vi "Retro.vi"(11 "Choose Directory":path) -> ()   [LabVIEW 2022 SP3]
uses:
  <vilib>/Analysis/NI_AALPro.lvlib
  <vilib>/Analysis/2dsp.llb/Complex FFT.vi
  <vilib>/Analysis/3filter.llb/Filter Passband Type.ctl
  <vilib>/Analysis/NI_AALBase.lvlib
  <vilib>/Analysis/3filter.llb/Butterworth Filter (DBL).vi
  <vilib>/Analysis/baseanly.llb/Quick Scale 1D.vi
  <vilib>/Analysis/baseanly.llb/Mean (DBL).vi
panel:
  in  "Save Directory":path
  out "Intensity Graph 3":sgl[][](graph)
  out "EKG 3":dbl[](graph)
  out "EKG 2":dbl[](graph)
  out "Intensity Graph 2":dbl[][](graph)
  in  "Use Selected Files":bool
  in  "Listbox":i32[](listbox)
  in  "file ext":string="000"
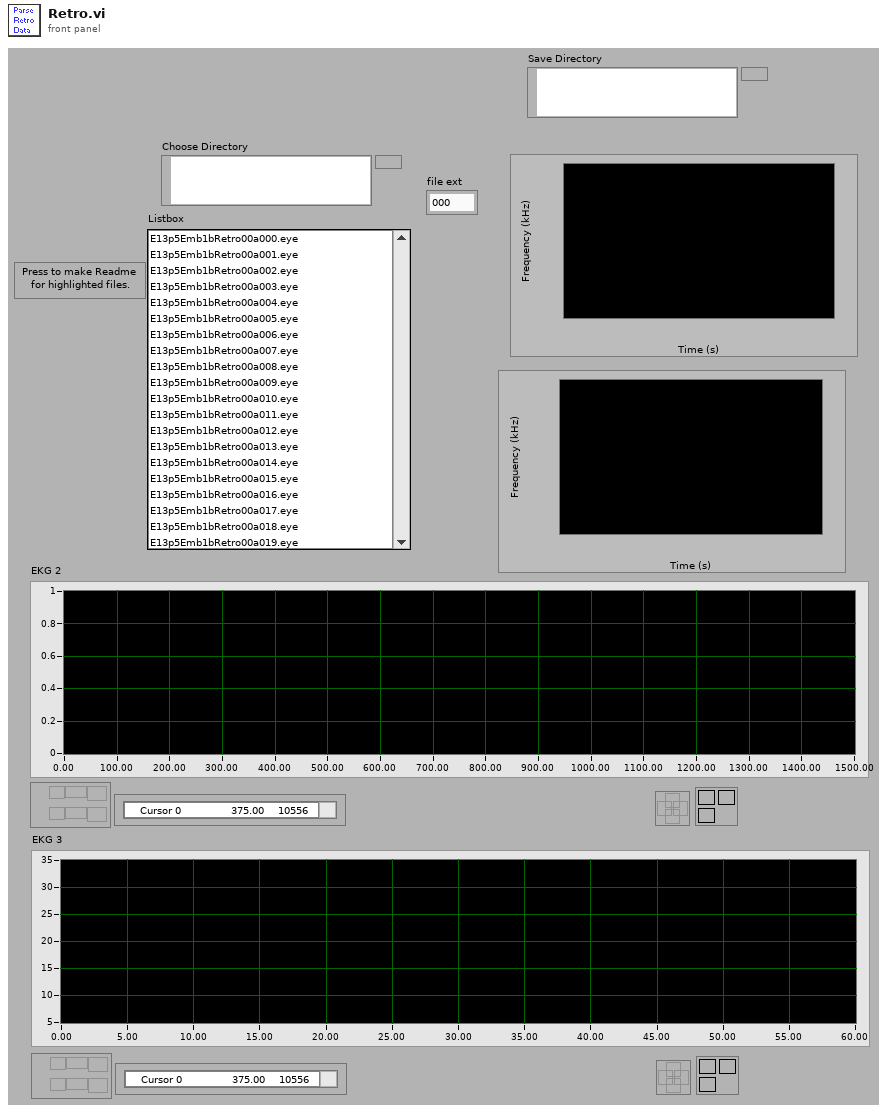
[diagram p1: front panel]
types:
  T1 = enum16{"big-endian, network order", "native, host order", "little-endian"}
  T2 = typedef "NI_AALBase.lvlib/Filter Passband Type.ctl" = enum32{"Lowpass", "Highpass", "Bandpass", "Bandstop"}
  T3 = enum16{"open", "replace", "create", "open or create", "replace or create", "replace or create with confirmation"}
  T4 = typedef "Header.ctl" = cluster{"header info":cluster{"Header":string, "Head length":i16}, "A/D info":cluster{"# rf points per line":u16, "# lines per scan":u16, "sample rate MHz":u16, "# A/D bits":i16, "# bytes per A/D":u16, "TGC Flag":u16, "A/D Type":string}, "Tranducer Info":cluster{"bandwidth":sgl, "center freq":sgl, "start freq":sgl, "ID":i32}, "Scan Info":cluster{"delay":sgl, "pivot distance":sgl, "sector scan angle":sgl, "operator":string, "Scan Mode":string, "location":string}, "Time/Date Info":cluster{"date":string, "time":string}, "RF Info":cluster{"RF file name":string, "RF file att":string, "RF cal file name":string, "RF cal file att":string}, "Patient Info":cluster{"ID":string, "extended ID":string, "age":u16, "sex":string, "previously\nscanned":string, "PSA":sgl, "LOS":u8, "Ethnicty 2":u8, "Race":u8}, "Tissue Type":cluster{"organ":i16, "disease type":i16, "disease location":i16}, "Votage scaling":cluster{"Digitizer (dB)":sgl, "Gain (dB)":sgl, "Atten (dB)":sgl}, "Comment":string, "Misc Info":cluster{"avg num":i16, "c speed":i16, "Div By or SF zones":i16, "XMIT CHS":u8, "RCV CHS":u8}, "Therapy Parameters":cluster{"Theraputic Freq (MHz)":sgl, "Time on (s)":sgl, "Therapy amplitude (mV)":sgl, "Lines Before":u16, "Lines After":u16}, "Scan Settings":cluster{"Energy (uJ or V)":u8, "Damp (Ohm) or Fc":u8, "HP Filt (KHz)":u8, "LP Filt (MHz)":u8, "Gain (db)":u8, "prf (kHz)":sgl, "Distance between\nscan lines (mm)":u16, "Distance between\nscan planes (mm)":u16}, "Compression Parameters":cluster{"F1 (MHz)":sgl, "F2 (MHz)":sgl, "% taper":sgl, "duration":sgl}, "Patient Info Xtra":cluster{"First Name":string, "Last Name":string, "Notes":string}}
  T5 = cluster{"Energy (uJ) or V":u8, "Damp (Ohm) or Fc":u8, "HP Filt(KHz) ":u8, "LP Filt (MHz)":u8, "Gain (db)":u8, "prf (kHz)":sgl, "Distance between\nscan lines (mm)":u16, "Distance between\nscan planes (mm)":u16}
  T6 = cluster{"# rf points per line":u16, "# lines per scan":u16, "sample rate MHz":u16, "# A/D bits":i16, "# bytes per A/D":u16, "TGC Flag":u16, "A/D Type":string}
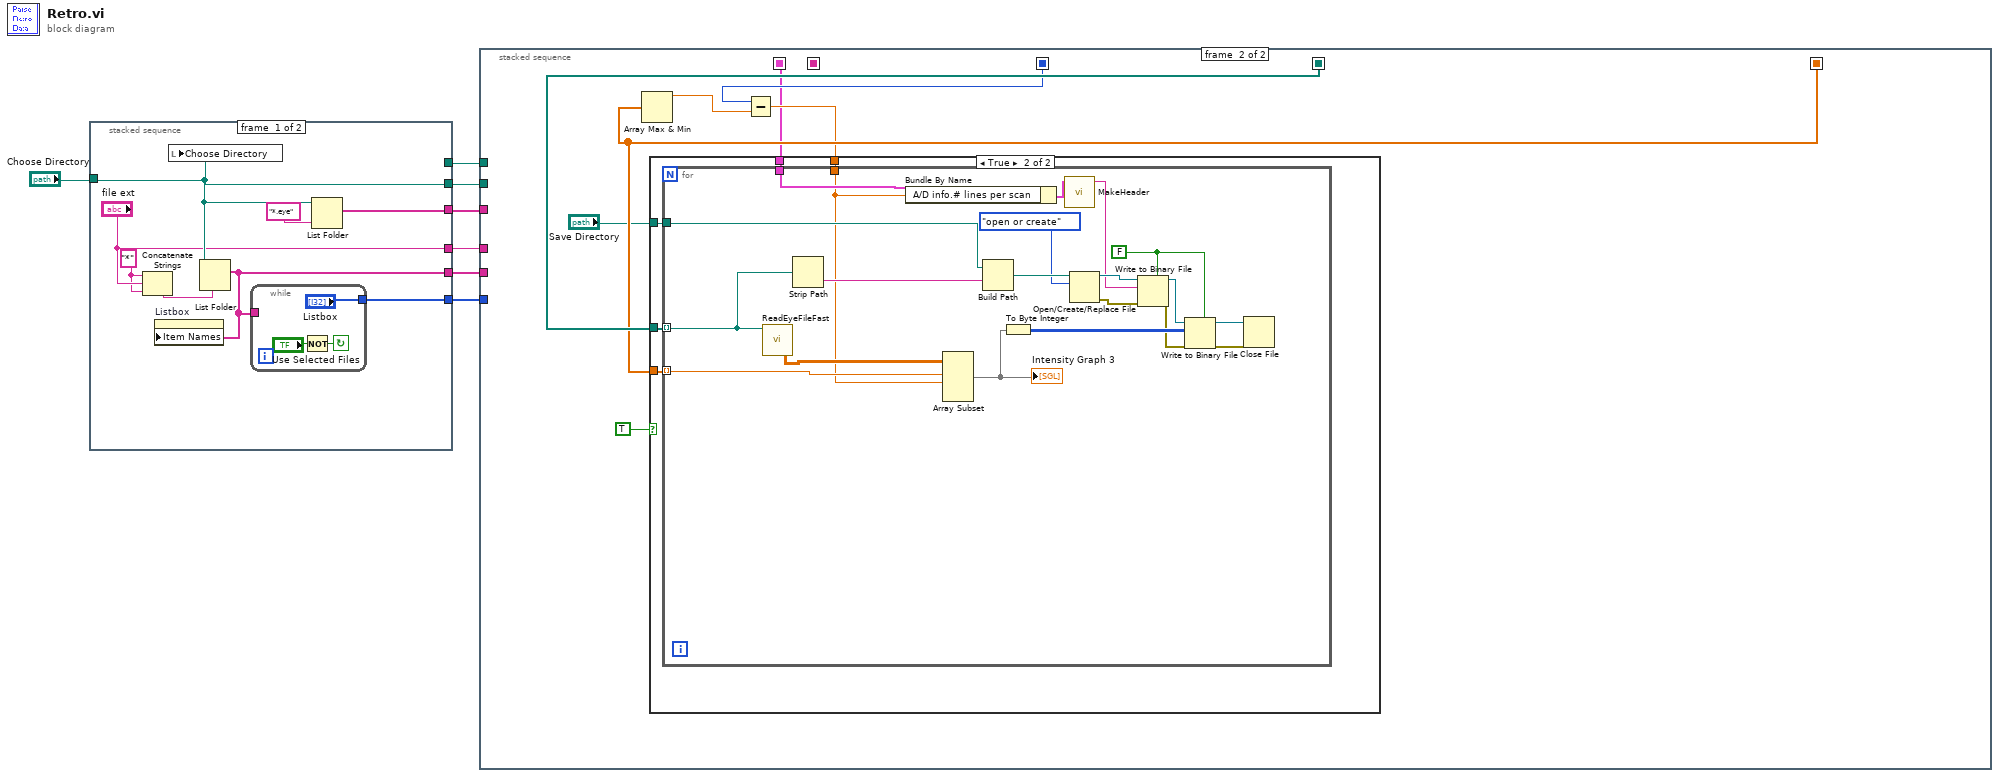
[diagram p0: block diagram]
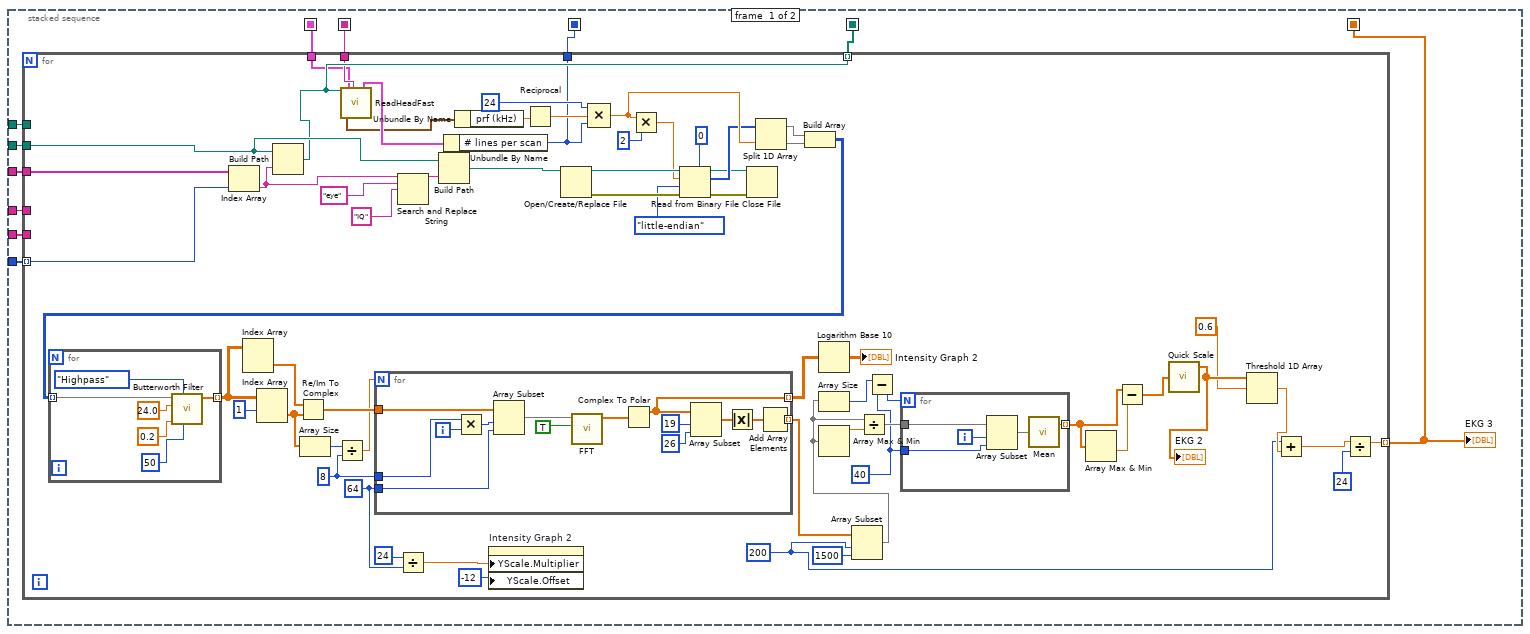
[diagram p2: hidden frame]
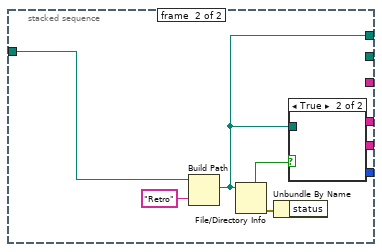
[diagram p4: hidden frame]
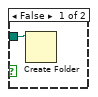
[diagram p5: hidden frame]
diagram:
  n1 = stacked-sequence {
    tunnel: "Choose Directory" -> [w11 w23]
    tunnel: [w14 _] -> w1
    tunnel: [w13 _] -> w6
    tunnel: [w12 _] -> w5
    tunnel: ["file ext" _] -> w4
    tunnel: [w11 _] -> w3
    tunnel: [_ w19] -> w2
    frame #0 {
      w8 = "*" ("prompt")
      n2 = Concatenate Strings(w8, "file ext", w8) -> (w9:string)
      n3 = local write "Choose Directory"(w11) -> ()
      n4 = List Folder(path=w11, pattern=w9) -> (filenames=w12:string[])  [unwired: 1 in, 4 out]
      n5 = property on="Listbox" class="LstBox (strict)"("Item Names"=w12) -> ()  [unwired: 2 in, 2 out]
      n6 = while {
        tunnel: ["Listbox"] -> w13
        tunnel: w12 -> [_]
        stop <- w18 continue-if-true
        n7 = Not(x="Use Selected Files") -> (.not. x?=w18:bool)
      }
      n8 = List Folder(path=w11, pattern="*.eye" ("prompt")) -> (filenames=w14:string[])  [unwired: 1 in, 4 out]
    }
    frame #1 {
      n9 = Build Path(base path=w23, name or relative path="Retro") -> (appended path=w19:path)
      n10 = File/Directory Info(path=w19) -> (directory=w21:bool, error out=w20:errorcluster)  [unwired: 1 in, 5 out]
      n11 = Unbundle By Name(w20) -> ()  [unwired: 1 out]
      n12 = case shown="True" w21 {
        tunnel: w19 -> [w24 _]
        frame False {
          n13 = Create Folder(path (use dialog)=w24) -> ()  [unwired: 1 in, 4 out]
        }
        frame True {
        }
      }
    }
  }
  n14 = stacked-sequence {
    seq-local: [w29 _] -> [_ w130]
    seq-local: [w28 _] -> [_ w129]
    seq-local: [w27 _] -> [_ w128]
    seq-local: [w26 _] -> [_ _]
    seq-local: [w25 _] -> [_ w123]
    tunnel: w6 -> [w35 _]
    tunnel: w5 -> [w34 _]
    tunnel: w4 -> [w33 _]
    tunnel: w3 -> [w32 _]
    tunnel: w2 -> [w31 _]
    tunnel: w1 -> [w30 _]
    frame #0 {
      n15 = for {
        tunnel: w35 -> [w77] mode=indexing
        tunnel: w34 -> [_]
        tunnel: w33 -> [_]
        tunnel: w32 -> [w74]
        tunnel: w31 -> [_]
        tunnel: w30 -> [w78]
        tunnel: [w51] -> w28 mode=indexing
        tunnel: [w55] -> w29 mode=indexing
        tunnel: [w54] -> w27
        tunnel: [w53] -> w26
        tunnel: [w42] -> w25
        w37 = 200
        w48 = 40
        w67 = 8
        w63 = 64
        n16 = Index Array(array=w78, index=w77) -> (element=w73:string)
        n17 = Build Path(base path=w74, name or relative path=w73) -> (appended path=w55:path)
        n18 = call "ReadHeadFast.vi"("new file path"=w55) -> ("Header In"=w42:T4, "Scan Settings (Pulser and Scaping)"=w75:T5, "raw header out"=w53:string, "A/D info"=w76:T6)  [unwired: 2 in, 13 out]
        n19 = Search and Replace String(input string=w73, search string="eye", replace string="IQ") -> (result string=w94:string)  [unwired: 1 in, 7 out]
        n20 = Divide(x=24, y=w63) -> (x/y=w62:dbl)
        n21 = Build Path(base path=w74, name or relative path=w94) -> (appended path=w95:path)
        n22 = Unbundle By Name(w76) -> ("# lines per scan"=w54:u16)
        n23 = Unbundle By Name(w75) -> ("prf (kHz)"=w79:sgl)
        n24 = property on="Intensity Graph 2" class="IntGraph (strict)"("YScale.Multiplier"=w62, "YScale.Offset"=-12) -> ()  [unwired: 2 in, 2 out]
        n25 = Reciprocal(x=w79) -> (1/x=w84:sgl)
        n26 = Open/Create/Replace File(file path (use dialog)=w95) -> (refnum out=w96:refnum<file>, error out=w97:errorcluster)  [unwired: 1 in, 5 out]
        n27 = Compound Arithmetic op=MULTIPLY(24, w84, w54) -> (w91:sgl)
        n28 = Multiply(x=w91, y=2) -> (x*y=w89:sgl)
        n29 = Read from Binary File(5:i16 0, 8:w97, 9:T1."little-endian" ("byte order (0:big-endian, network order)"), 10:w89, 11:w96) -> (0:w81:errorcluster, 2:w88:i16[], 3:w82:refnum<file>)  [unwired: 2 out]
        n30 = Close File(refnum=w82, error in=w81) -> ()  [unwired: 2 out]
        n31 = Split 1D Array(array=w88, index=w91) -> (first subarray=w92:i16[], second subarray=w93:i16[])
        n32 = Build Array(w92, w93) -> (w56:i16[][])
        n33 = for {
          tunnel: w56 -> [w103] mode=indexing
          tunnel: [w102] -> w57 mode=indexing
          n34 = call-poly <vilib>:"Butterworth Filter.vi"("order"=50, "filter type"=Filter_Passband_Type."Highpass", "low cutoff freq: fl"=0.2, "sampling freq: fs"=24.0, "X"=w103) -> ("Filtered X"=w102:dbl[])  [unwired: 3 in, 1 out]
        }
        n35 = Index Array(array=w57) -> (element=w68:dbl[])  [unwired: 2 in]
        n36 = Index Array(array=w57, index (row)=1) -> (element=w69:dbl[])  [unwired: 1 in]
        n37 = Re/Im To Complex(1:w69, 2:w68) -> (0:w70:cdb[])
        n38 = Array Size(array=w69) -> (size(s)=w71:i32)
        n39 = Divide(x=w71, y=w67) -> (x/y=w66:dbl)
        n40 = for {
          N: w66 -> [_]
          tunnel: w70 -> [w122]
          tunnel: w63 -> [w110]
          tunnel: w67 -> [w120]
          tunnel: [w113] -> w61 mode=indexing
          tunnel: [w114] -> w41 mode=indexing
          i -> [w121]
          n41 = Multiply(x=w120, y=w121) -> (x*y=w119:i32)
          n42 = Array Subset(array=w122, index=w119, length=w110) -> (w118:cdb[])
          n43 = call-poly <vilib>:"FFT.vi"("shift?"=TRUE, "X"=w118) -> ("FFT {X}"=w116:cdb[])  [unwired: 8 in, 1 out]
          n44 = Complex To Polar(r * e^(i*theta)=w116) -> (r=w113:dbl[])  [unwired: 1 out]
          n45 = Array Subset(array=w113, index=19, length=26) -> (w112:dbl[])
          n46 = Absolute Value(x=w112) -> (abs(x)=w115:dbl[])
          n47 = Add Array Elements(numeric array=w115) -> (sum=w114:dbl)
        }
        n48 = Logarithm Base 10(1:w61) -> (0:→"Intensity Graph 2":dbl[][])
        n49 = Array Subset(array=w41, index=w37, length=1500) -> (w40:dbl[])
        n50 = Array Size(array=w40) -> (size(s)=w49:i32)
        n51 = Array Max & Min(array=w40) -> (max value=w59:dbl)  [unwired: 3 out]
        n52 = Divide(x=w40, y=w59) -> (x/y=w58:dbl[])
        n53 = Subtract(x=w49, y=w48) -> (x-y=w50:i32)
        n54 = for {
          N: w50 -> [_]
          tunnel: w58 -> [w108]
          tunnel: [w105] -> w46 mode=indexing
          tunnel: w48 -> [w104]
          i -> [w106]
          n55 = Array Subset(array=w108, index=w106, length=w104) -> (w107:dbl[])
          n56 = call-poly <vilib>:"Mean.vi"("X"=w107) -> ("mean"=w105:dbl)  [unwired: 1 out]
        }
        n57 = Array Max & Min(array=w46) -> (min value=w47:dbl)  [unwired: 3 out]
        n58 = Subtract(x=w46, y=w47) -> (x-y=w45:dbl[])
        n59 = call-poly <vilib>:"Quick Scale.vi"("X"=w45) -> ("Y[i]=X[i]/Max|X|"=w44:dbl[])  [unwired: 2 out]
        "EKG 2" <- w44
        n60 = Threshold 1D Array(2:0.6 ("threshold"), 3:w44) -> (0:w38:dbl)  [unwired: 1 in]
        n61 = Add(x=w37, y=w38) -> (x+y=w36:dbl)
        n62 = Divide(x=w36, y=24) -> (x/y=w51:dbl)
      }
      "EKG 3" <- w28
    }
    frame #1 {
      n63 = Array Max & Min(array=w129) -> (max value=w127:dbl)  [unwired: 3 out]
      n64 = Subtract(x=w128, y=w127) -> (x-y=w126:dbl)
      n65 = case shown="True" TRUE {
        tunnel: w130 -> [_ w135]
        tunnel: w129 -> [_ w134]
        tunnel: w126 -> [_ w133]
        tunnel: "Save Directory" -> [_ w132]
        tunnel: w123 -> [_ w131]
        frame False {
        }
        frame True {
          n66 = for {
            tunnel: w135 -> [w153] mode=indexing
            tunnel: w134 -> [w154] mode=indexing
            tunnel: w133 -> [w136]
            tunnel: w132 -> [w151]
            tunnel: w131 -> [w139]
            w141 = FALSE ("prepend array or string size? (T)")
            n67 = call "ReadEyeFileFast.vi"("new file path"=w153) -> ("2-D data array"=w155:sgl[][])  [unwired: 1 in, 17 out]
            n68 = Strip Path(path=w153) -> (name=w152:string)  [unwired: 1 out]
            n69 = Bundle By Name(cluster=w139, "A/D info.# lines per scan"=w136) -> (w138:T4)
            n70 = Array Subset(array=w155, index (row)=w154, length (row)=w136) -> (w149:sgl[][])  [unwired: 2 in]
            "Intensity Graph 3" <- w149
            n71 = Build Path(base path=w151, name or relative path=w152) -> (appended path=w150:path)
            n72 = To Byte Integer(number=w149) -> (8bit integer=w148:i8[][])
            n73 = call "MakeHeader.vi"("Header In"=w138) -> ("Header String"=w137:string)  [unwired: 6 out]
            n74 = Open/Create/Replace File(file path (use dialog)=w150, operation (0:open)=T3."open or create") -> (refnum out=w147:refnum<file>, error out=w145:errorcluster)  [unwired: 4 in, 1 out]
            n75 = Write to Binary File(file (use dialog)=w147, data=w137, error in=w145, 5:w141) -> (refnum out=w146:refnum<file>, error out=w144:errorcluster)  [unwired: 2 in, 1 out]
            n76 = Write to Binary File(file (use dialog)=w146, data=w148, error in=w144, 5:w141) -> (refnum out=w142:refnum<file>, error out=w143:errorcluster)  [unwired: 2 in, 1 out]
            n77 = Close File(refnum=w142, error in=w143) -> ()  [unwired: 2 out]
          }
        }
      }
    }
  }
